vi "Teleskop_Optotune.vi"() -> ()   [LabVIEW 2013]
uses:
  Hello Optotune Lens (30.06.2014)/Calibration.ctl
  <vilib>/Instr/_visa.llb/VISA Configure Serial Port (Instr).vi
panel:
  out "D2":dbl
  out "D1":dbl
  out "I_var_2":dbl=-2.842170943040401e-14
  out "I_var_1":dbl=294.1354035926154
  out "M":dbl=2.502800028000281
  out "f_2":dbl=79.93605052008911
  out "f_1":dbl=200.0639494799109
  in  "Vergrößerung":dbl(slide)=10.0 scale=0.0..10.0
  out "M_min":dbl=0.39955249672863113
  out "M_max":dbl=2.5028000280002805
  out "f_1_max_real":dbl=200.0639494799109
  out "f_2_max_real":dbl=200.0639494799109
  in  "Eigener Abstand e":dbl=280.0 format="%#_13g"
  out "Vorgeschlagener Abstand Linsen e":dbl=71507.79319337723
  in  "f_offset 2":dbl=99999.0
  out "f_2_min":dbl=79.93605052008913
  out "f_2_max":dbl=71427.85714285714
  out "f_1_min":dbl=79.93605052008913
  out "f_1_max":dbl=71427.85714285714
  in  "f_min":dbl=80.0
  in  "f_offset 1":dbl=99999.0
  in  "f_max":dbl=200.0
  out "I_max":dbl
  out "I_min":dbl
  out "VISA resource name out 2":string="COM13"
  out "Calibration 3":T1={"Max Current A"=292.84, "Max Current B"=293.0, "UCL A"=292.76850585937495, "UCL B"=300.0, "LCL A"=4392.671494140624, "LCL B"=0.0} {"Max Current A" format="%#_g mA"; "Max Current B" format="%#_g mA"; "UCL A" format="%#_g mA"; "LCL A" format="%#_g mA"; "UCL B" format="%#_g mA"; "LCL B" format="%#_g mA"}
  out "OK 2":bool=TRUE
  out "Data 2":string
  out "Current Ch A (mA) 2":dbl=-2.842170943040401e-14
  out "Command to Port 2":string
  out "TA (°C) 2":dbl
  in  "Read Temperature 2":bool caption="Send Command"
  out "ID 2":u16
  in  "Calibration 4":T1={"Max Current A"=293.0, "Max Current B"=293.0, "UCL A"=300.0, "UCL B"=300.0, "LCL A"=0.0, "LCL B"=0.0} {"Max Current A" format="%#_g mA"; "Max Current B" format="%#_g mA"; "UCL A" format="%#_g mA"; "LCL A" format="%#_g mA"; "UCL B" format="%#_g mA"; "LCL B" format="%#_g mA"}
  out "error out 2":errorcluster={"status"=FALSE, "code"=1073676294, "source"="VISA Read in write read Lens Driver.vi->Teleskop_Optotune.vi"}
  in  "error in (no error) 2":errorcluster
  in  "VISA resource name 2":string="COM13"
  in  "Calibration":T1={"Max Current A"=293.0, "Max Current B"=293.0, "UCL A"=300.0, "UCL B"=300.0, "LCL A"=0.0, "LCL B"=0.0} {"Max Current A" format="%#_g mA"; "Max Current B" format="%#_g mA"; "UCL A" format="%#_g mA"; "LCL A" format="%#_g mA"; "UCL B" format="%#_g mA"; "LCL B" format="%#_g mA"}
  out "ID":u16
  in  "stop":bool
  out "VISA resource name out":string="COM14"
  out "Calibration 2":T1={"Max Current A"=292.84, "Max Current B"=293.0, "UCL A"=292.76850585937495, "UCL B"=300.0, "LCL A"=4392.671494140624, "LCL B"=0.0} {"Max Current A" format="%#_g mA"; "Max Current B" format="%#_g mA"; "UCL A" format="%#_g mA"; "LCL A" format="%#_g mA"; "UCL B" format="%#_g mA"; "LCL B" format="%#_g mA"}
  out "OK":bool=TRUE
  out "Data":string
  out "Current Ch A (mA)":dbl=294.1354035926154
  out "Command to Port":string
  out "TA (°C)":dbl
  in  "Read Temperature":bool caption="Send Command"
  out "error out":errorcluster={"status"=FALSE, "code"=1073676294, "source"="VISA Read in write read Lens Driver.vi->Teleskop_Optotune.vi"}
  in  "error in (no error)":errorcluster
  in  "VISA resource name":string="COM14"
  # "Parameter Teleskop:"
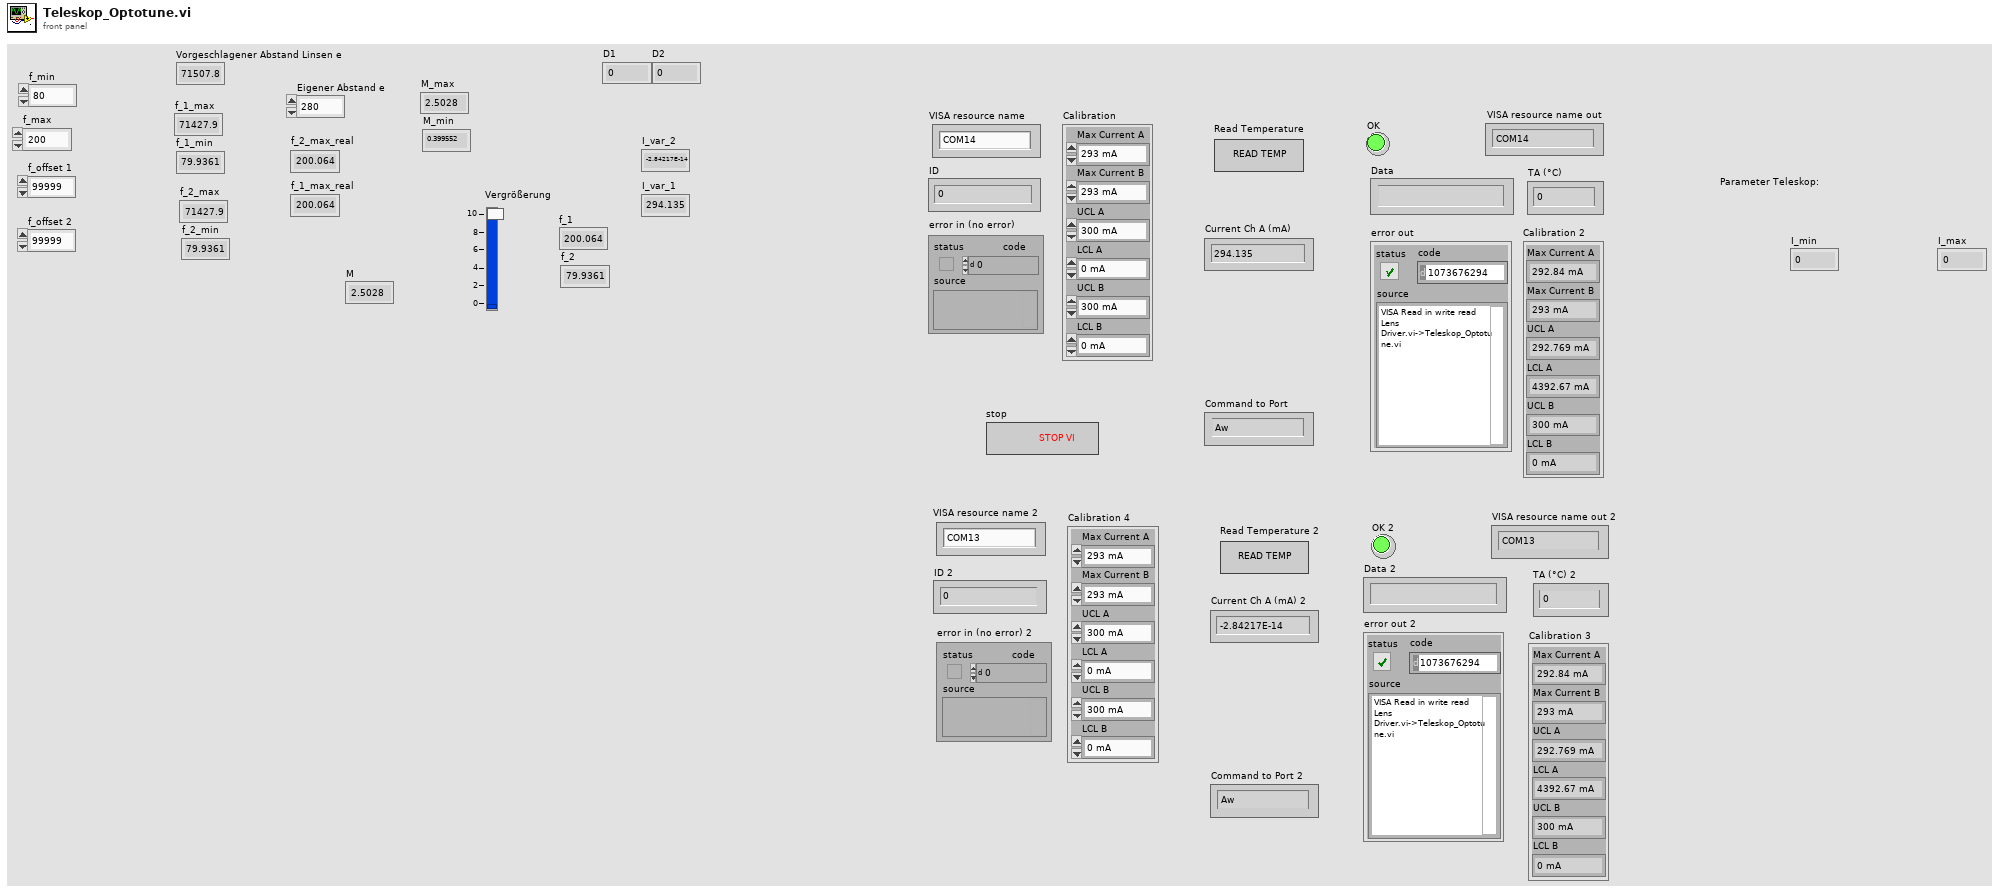
[diagram p1: front panel]
types:
  T1 = typedef "Calibration.ctl" = cluster{"Max Current A":dbl, "Max Current B":dbl, "UCL A":dbl, "UCL B":dbl, "LCL A":dbl, "LCL B":dbl}
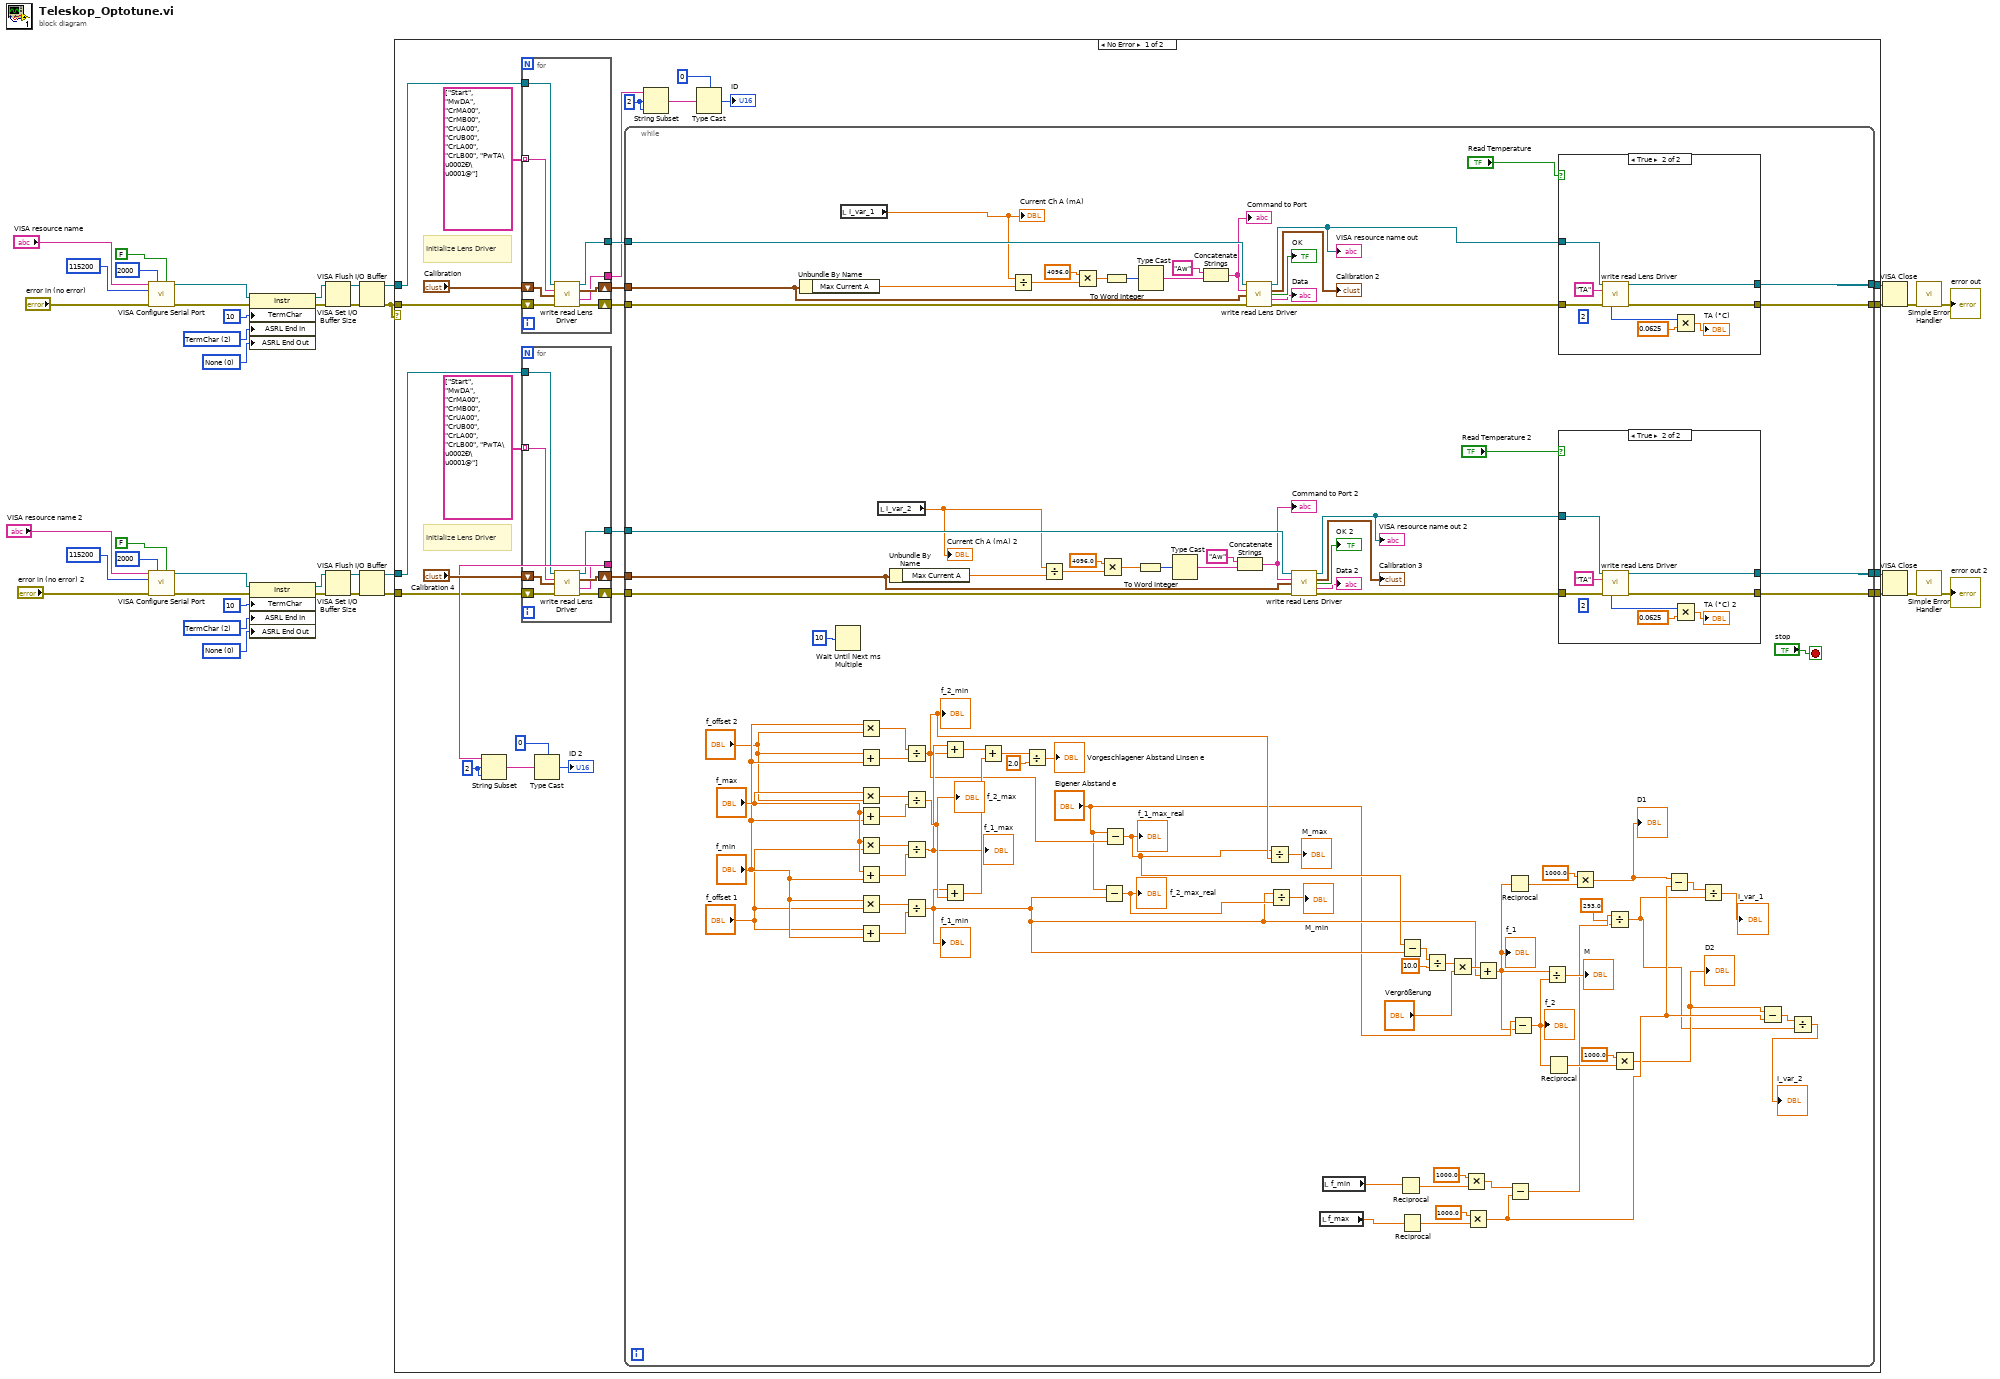
[diagram p0: block diagram]
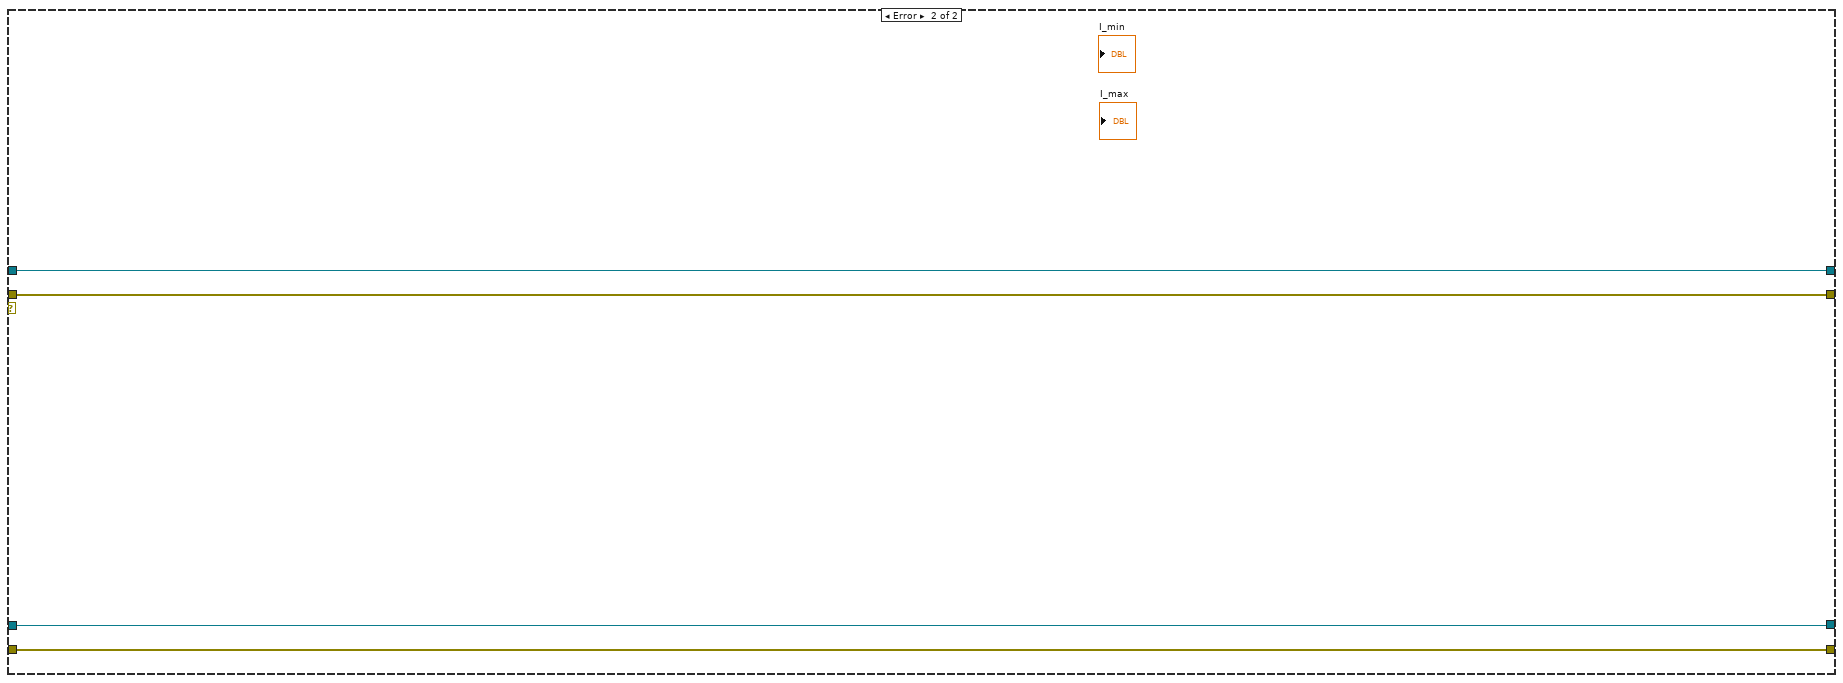
[diagram p4: hidden frame]
diagram:
  w11 = u16 0 items=["None", "Last Bit", "TermChar", "Break"] ("Serial Settings:End Mode for Writes")
  w12 = u16 2 items=["None", "Last Bit", "TermChar"] ("Serial Settings:End Mode for Reads")
  w31 = u16 0 items=["None", "Last Bit", "TermChar", "Break"] ("Serial Settings:End Mode for Writes")
  w32 = u16 2 items=["None", "Last Bit", "TermChar"] ("Serial Settings:End Mode for Reads")
  n1 = call-poly "VISA Configure Serial Port"("VISA resource name"="VISA resource name", "timeout (10sec)"=u32 2000, "Enable Termination\nChar (T)"=FALSE ("Enable Termination\nChar (T)"), "baud rate (9600)"=u32 115200, "error in (no error)"="error in (no error)") -> ("VISA resource name out"=w36:refnum<visa-resource-name>, "error out"=w34:errorcluster)  [unwired: 9 in]
  n2 = call-poly "VISA Configure Serial Port"("VISA resource name"="VISA resource name 2", "timeout (10sec)"=u32 2000, "Enable Termination\nChar (T)"=FALSE ("Enable Termination\nChar (T)"), "baud rate (9600)"=u32 115200, "error in (no error)"="error in (no error) 2") -> ("VISA resource name out"=w16:refnum<visa-resource-name>, "error out"=w14:errorcluster)  [unwired: 9 in]
  n3 = property class="Instr"(reference=w36, error in=w34, "TermChar"=u8 10 ("Message Based Settings:Termination Character"), "ASRL End In"=w32, "ASRL End Out"=w31) -> (reference out=w35:refnum<visa-resource-name>, error out=w33:errorcluster)
  n4 = property class="Instr"(reference=w16, error in=w14, "TermChar"=u8 10 ("Message Based Settings:Termination Character"), "ASRL End In"=w12, "ASRL End Out"=w11) -> (reference out=w15:refnum<visa-resource-name>, error out=w13:errorcluster)
  n5 = VISA Set I/O Buffer Size(VISA resource name=w35, error in (no error)=w33) -> (VISA resource name out=w28:refnum<visa-resource-name>, error out=w27:errorcluster)  [unwired: 2 in]
  n6 = VISA Set I/O Buffer Size(VISA resource name=w15, error in (no error)=w13) -> (VISA resource name out=w8:refnum<visa-resource-name>, error out=w7:errorcluster)  [unwired: 2 in]
  n7 = VISA Flush I/O Buffer(VISA resource name=w28, error in (no error)=w27) -> (VISA resource name out=w26:refnum<visa-resource-name>, error out=w21:errorcluster)  [unwired: 1 in]
  n8 = VISA Flush I/O Buffer(VISA resource name=w8, error in (no error)=w7) -> (VISA resource name out=w4:refnum<visa-resource-name>, error out=w3:errorcluster)  [unwired: 1 in]
  n9 = case shown="No Error" w21 {
    tunnel: w21 -> [w68 w204]
    tunnel: w26 -> [w67 w205]
    tunnel: [w66 w204] -> w24
    tunnel: [w65 w205] -> w22
    tunnel: w4 -> [w46 w203]
    tunnel: w3 -> [w45 w202]
    tunnel: [w42 w203] -> w2
    tunnel: [w41 w202] -> w1
    frame No Error {
      w53 = 2 ("length (rest)")
      w63 = 2 ("length (rest)")
      # "Initialize Lens Driver"
      # "Initialize Lens Driver"
      n10 = for {
        tunnel: w67 -> [w200]
        tunnel: [w197] -> w57
        tunnel: string[] ["Start", "MwDA", "CrMA00", "CrMB00", "CrUA00", "CrUB00", "CrLA00", "CrLB00", "PwTA\u0002Ð\u0001@"] -> [w195] mode=indexing
        tunnel: [w194] -> w56
        shift-right: [w198] -> w58
        shift-left: "Calibration" -> [w199]
        shift-right: [w196] -> w59
        shift-left: w68 -> [w201]
        n11 = call "write read Lens Driver.vi"("VISA resource name"=w200, "command"=w195, "Calibration"=w199, "error in (no error)"=w201) -> ("VISA resource name out"=w197:refnum<visa-resource-name>, "Calibration 2"=w198:T1, "Data"=w194:string, "error out"=w196:errorcluster)  [unwired: 4 in, 4 out]
      }
      n12 = for {
        tunnel: w46 -> [w192]
        tunnel: [w189] -> w48
        tunnel: string[] ["Start", "MwDA", "CrMA00", "CrMB00", "CrUA00", "CrUB00", "CrLA00", "CrLB00", "PwTA\u0002Ð\u0001@"] -> [w187] mode=indexing
        tunnel: [w186] -> w47
        shift-right: [w190] -> w49
        shift-left: "Calibration 4" -> [w191]
        shift-right: [w188] -> w50
        shift-left: w45 -> [w193]
        n13 = call "write read Lens Driver.vi"("VISA resource name"=w192, "command"=w187, "Calibration"=w191, "error in (no error)"=w193) -> ("VISA resource name out"=w189:refnum<visa-resource-name>, "Calibration 2"=w190:T1, "Data"=w186:string, "error out"=w188:errorcluster)  [unwired: 4 in, 4 out]
      }
      n14 = String Subset(string=w47, offset (0)=w53, length (rest)=w53) -> (substring=w51:string)
      n15 = Type Cast(type=u16 0 ("length (rest)"), x=w51) -> (*(type *) &x=→"ID 2":u16)
      n16 = while {
        tunnel: [w165] -> w66
        tunnel: [w164] -> w65
        tunnel: w59 -> [w163]
        tunnel: w58 -> [w162]
        tunnel: w57 -> [w161]
        tunnel: w50 -> [w160]
        tunnel: w49 -> [w159]
        tunnel: w48 -> [w158]
        tunnel: [w149] -> w42
        tunnel: [w148] -> w41
        stop <- "stop" stop-if-true
        n17 = Unbundle By Name(w162) -> ("Max Current A"=w93:dbl)
        n18 = Wait Until Next ms Multiple(millisecond multiple=u32 10) -> ()  [unwired: 1 out]
        n19 = local read "I_var_1"() -> (w92:dbl)
        "Current Ch A (mA)" <- w92
        n20 = Multiply(x="f_min", y="f_offset 2") -> (x*y=w142:dbl)
        n21 = Add(x="f_offset 2", y="f_min") -> (x+y=w143:dbl)
        n22 = Multiply(x="f_max", y="f_offset 2") -> (x*y=w140:dbl)
        n23 = Add(x="f_max", y="f_min") -> (x+y=w141:dbl)
        n24 = Multiply(x="f_max", y="f_offset 1") -> (x*y=w144:dbl)
        n25 = Add(x="f_max", y="f_min") -> (x+y=w145:dbl)
        n26 = Multiply(x="f_min", y="f_offset 1") -> (x*y=w146:dbl)
        n27 = Add(x="f_offset 1", y="f_min") -> (x+y=w147:dbl)
        n28 = local read "I_var_2"() -> (w104:dbl)
        "Current Ch A (mA) 2" <- w104
        n29 = Unbundle By Name(w159) -> ("Max Current A"=w105:dbl)
        n30 = Divide(x=w142, y=w143) -> (x/y=w129:dbl)
        "f_2_min" <- w129
        n31 = Divide(x=w140, y=w141) -> (x/y=w132:dbl)
        "f_2_max" <- w132
        n32 = Divide(x=w144, y=w145) -> (x/y=w131:dbl)
        "f_1_max" <- w131
        n33 = Divide(x=w146, y=w147) -> (x/y=w120:dbl)
        "f_1_min" <- w120
        n34 = Add(x=w131, y=w129) -> (x+y=w136:dbl)
        n35 = Add(x=w120, y=w132) -> (x+y=w135:dbl)
        n36 = Add(x=w136, y=w135) -> (x+y=w134:dbl)
        n37 = Divide(x=w92, y=w93) -> (x/y=w100:dbl)
        n38 = Divide(x=w134, y=2.0) -> (x/y=→"Vorgeschlagener Abstand Linsen e":dbl)
        n39 = Divide(x=w104, y=w105) -> (x/y=w112:dbl)
        n40 = Multiply(x=4096.0, y=w100) -> (x*y=w98:dbl)
        n41 = Multiply(x=4096.0, y=w112) -> (x*y=w110:dbl)
        n42 = Subtract(x="Eigener Abstand e", y=w120) -> (x-y=w130:dbl)
        "f_2_max_real" <- w130
        n43 = Subtract(x="Eigener Abstand e", y=w129) -> (x-y=w126:dbl)
        "f_1_max_real" <- w126
        n44 = To Word Integer(number=w98) -> (16bit integer=w97:i16)
        n45 = To Word Integer(number=w110) -> (16bit integer=w109:i16)
        n46 = Type Cast(x=w97) -> (*(type *) &x=w96:string)  [unwired: 1 in]
        n47 = Type Cast(x=w109) -> (*(type *) &x=w108:string)  [unwired: 1 in]
        n48 = Concatenate Strings("Aw", w96) -> (w94:string)
        "Command to Port" <- w94
        n49 = Concatenate Strings("Aw", w108) -> (w106:string)
        "Command to Port 2" <- w106
        n50 = call "write read Lens Driver.vi"("VISA resource name"=w161, "command"=w94, "Calibration"=w162, "error in (no error)"=w163) -> ("VISA resource name out"=w153:refnum<visa-resource-name>, "Calibration 2"=→"Calibration 2":T1, "OK"=→"OK":bool, "Data"=→"Data":string, "error out"=w152:errorcluster)  [unwired: 4 in, 3 out]
        "VISA resource name out" <- w153
        n51 = Divide(x=w126, y=w129) -> (x/y=→"M_max":dbl)
        n52 = Divide(x=w120, y=w130) -> (x/y=→"M_min":dbl)
        n53 = call "write read Lens Driver.vi"("VISA resource name"=w158, "command"=w106, "Calibration"=w159, "error in (no error)"=w160) -> ("VISA resource name out"=w157:refnum<visa-resource-name>, "Calibration 2"=→"Calibration 3":T1, "OK"=→"OK 2":bool, "Data"=→"Data 2":string, "error out"=w156:errorcluster)  [unwired: 4 in, 3 out]
        "VISA resource name out 2" <- w157
        n54 = local read "f_max"() -> (w80:dbl)
        n55 = local read "f_min"() -> (w83:dbl)
        n56 = Reciprocal(x=w83) -> (1/x=w85:dbl)
        n57 = Subtract(x=w126, y=w120) -> (x-y=w125:dbl)
        n58 = Reciprocal(x=w80) -> (1/x=w82:dbl)
        n59 = Divide(x=w125, y=10.0) -> (x/y=w123:dbl)
        n60 = Multiply(x=w123, y="Vergrößerung") -> (x*y=w121:dbl)
        n61 = Multiply(x=1000.0, y=w85) -> (x*y=w79:dbl)
        n62 = Multiply(x=1000.0, y=w82) -> (x*y=w75:dbl)
        n63 = Add(x=w121, y=w120) -> (x+y=w90:dbl)
        "f_1" <- w90
        n64 = Reciprocal(x=w90) -> (1/x=w89:dbl)
        n65 = Subtract(x=w79, y=w75) -> (x-y=w70:dbl)
        n66 = Subtract(x="Eigener Abstand e", y=w90) -> (x-y=w91:dbl)
        "f_2" <- w91
        n67 = Divide(x=w90, y=w91) -> (x/y=→"M":dbl)
        n68 = Reciprocal(x=w91) -> (1/x=w86:dbl)
        n69 = case shown="True" "Read Temperature" {
          tunnel: [w167 w175] -> w164
          tunnel: [w166 w174] -> w165
          tunnel: w153 -> [w167 w173]
          tunnel: w152 -> [w166 w172]
          frame False {
          }
          frame True {
            (unwired) 2 ("length (rest)")
            n70 = call "write read Lens Driver.vi"("VISA resource name"=w173, "command"="TA", "error in (no error)"=w172) -> ("VISA resource name out"=w175:refnum<visa-resource-name>, "TA"=w169:u16, "error out"=w174:errorcluster)  [unwired: 5 in, 5 out]
            n71 = Multiply(x=w169, y=0.0625) -> (x*y=→"TA (°C)":dbl)
          }
        }
        n72 = case shown="True" "Read Temperature 2" {
          tunnel: [w177 w185] -> w149
          tunnel: [w176 w184] -> w148
          tunnel: w157 -> [w177 w183]
          tunnel: w156 -> [w176 w182]
          frame False {
          }
          frame True {
            (unwired) 2 ("length (rest)")
            n73 = call "write read Lens Driver.vi"("VISA resource name"=w183, "command"="TA", "error in (no error)"=w182) -> ("VISA resource name out"=w185:refnum<visa-resource-name>, "TA"=w179:u16, "error out"=w184:errorcluster)  [unwired: 5 in, 5 out]
            n74 = Multiply(x=w179, y=0.0625) -> (x*y=→"TA (°C) 2":dbl)
          }
        }
        n75 = Multiply(x=1000.0, y=w89) -> (x*y=w78:dbl)
        "D1" <- w78
        n76 = Divide(x=w70, y=293.0 ("x")) -> (x/y=w72:dbl)
        n77 = Multiply(x=1000.0, y=w86) -> (x*y=w74:dbl)
        "D2" <- w74
        n78 = Subtract(x=w78, y=w75) -> (x-y=w77:dbl)
        n79 = Divide(x=w77, y=w72) -> (x/y=→"I_var_1":dbl)
        n80 = Subtract(x=w74, y=w75) -> (x-y=w73:dbl)
        n81 = Divide(x=w73, y=w72) -> (x/y=→"I_var_2":dbl)
      }
      n82 = String Subset(string=w56, offset (0)=w63, length (rest)=w63) -> (substring=w61:string)
      n83 = Type Cast(type=u16 0 ("length (rest)"), x=w61) -> (*(type *) &x=→"ID":u16)
    }
    frame Error {
    }
  }
  n84 = VISA Close(VISA resource name=w22, error in (no error)=w24) -> (error out=w25:errorcluster)
  n85 = VISA Close(VISA resource name=w2, error in (no error)=w1) -> (error out=w6:errorcluster)
  n86 = call <vilib>:"Simple Error Handler.vi"("error in (no error)"=w25) -> ("error out"=→"error out":errorcluster)  [unwired: 4 in, 4 out]
  n87 = call <vilib>:"Simple Error Handler.vi"("error in (no error)"=w6) -> ("error out"=→"error out 2":errorcluster)  [unwired: 4 in, 4 out]
